vi "MB director next device.vi"(7 "New cmd":bool[](array[boolean])) -> (2 "Next priority index":i32, 3 "same index":bool)   [LabVIEW 2019]
panel:
  out "rotated array":bool[](array[boolean])
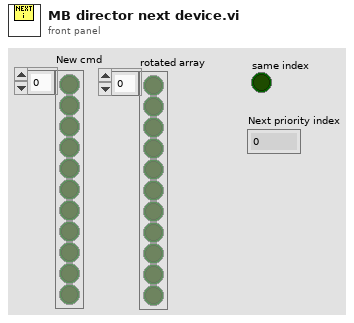
[diagram p1: front panel]
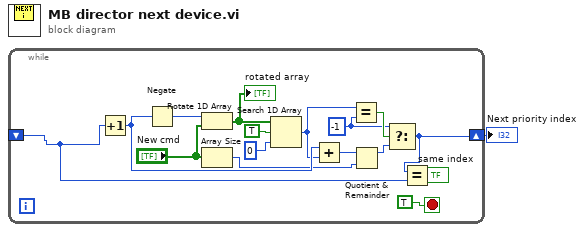
[diagram p0: block diagram]
diagram:
  n1 = while {
    shift-right: [w4] -> w1
    shift-left: _ -> [w3]
    stop <- TRUE stop-if-true
    w5 = -1 ("t")
    n2 = Increment(x=w3) -> (x+1=w11:i32)
    n3 = Negate(x=w11) -> (-x=w15:i32)
    n4 = Rotate 1D Array(1:"New cmd", 2:w15) -> (0:w16:bool[])
    "rotated array" <- w16
    n5 = Array Size(array="New cmd") -> (size(s)=w8:i32)
    n6 = Search 1D Array(1D array=w16, element=TRUE, start index (0)=0) -> (index of element=w9:i32)
    n7 = Add(x=w11, y=w9) -> (x+y=w13:i32)
    n8 = Equal?(x=w9, y=w5) -> (x = y?=w6:bool)
    n9 = Quotient & Remainder(x=w13, y=w8) -> (x-y*floor(x/y)=w7:i32)  [unwired: 1 out]
    n10 = Select(t=w5, s=w6, f=w7) -> (s? t:f=w4:i32)
    n11 = Equal?(x=w4, y=w3) -> (x = y?=→"same index":bool)
  }
  "Next priority index" <- w1
